vi "Populate Ctrl.vi"(8 "error in (no error)":errorcluster, 11 "Ctrl Refnum Column in":refnum<class "Ctrl Refnum Column.lvclass">) -> (0 "error out":errorcluster, 3 "Ctrl Refnum Column out":refnum<class "Ctrl Refnum Column.lvclass">)   [LabVIEW 2020, in "Basic Fields.lvlib" / "Ctrl Refnum Column.lvclass"]
uses:
  Ctrl Refnum Column.lvclass
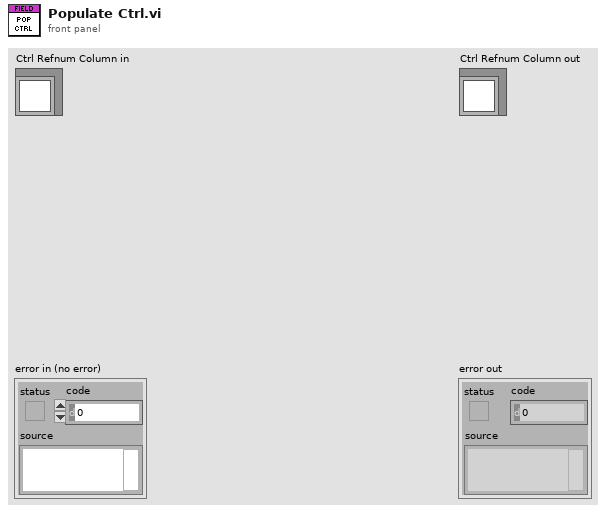
[diagram p1: front panel]
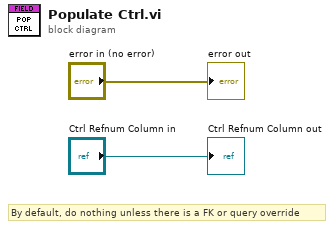
[diagram p0: block diagram]
diagram:
  # "By default, do nothing unless there is a FK or query override"
  "error out" <- "error in (no error)"
  "Ctrl Refnum Column out" <- "Ctrl Refnum Column in"
